vi "Test_Stage_Movement.vi"() -> ()   [LabVIEW 2013]
panel:
  in  "Numeric":dbl
  in  "Serial":i32=90848557
  in  "MG17Motor":refnum<k7>(container)
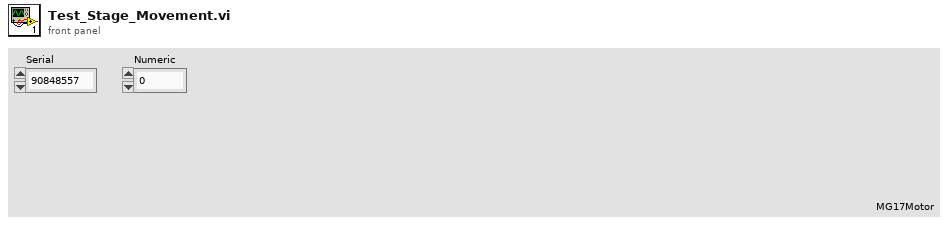
[diagram p1: front panel]
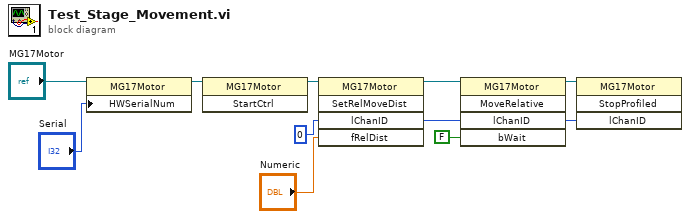
[diagram p0: block diagram]
diagram:
  n1 = property class="MG17Motor"(reference="MG17Motor", "HWSerialNum"="Serial") -> (reference out=w9:refnum<k7>)  [unwired: 1 in, 1 out]
  n2 = invoke class="MG17Motor" method="StartCtrl"(reference=w9) -> (reference out=w3:refnum<k7>)  [unwired: 2 in, 2 out]
  n3 = invoke class="MG17Motor" method="SetRelMoveDist"(reference=w3, "lChanID"=0, "fRelDist"="Numeric") -> (reference out=w7:refnum<k7>, "lChanID"=w6:i32)  [unwired: 2 in, 3 out]
  n4 = invoke class="MG17Motor" method="MoveRelative"(reference=w7, "lChanID"=w6, "bWait"=FALSE) -> (reference out=w5:refnum<k7>, "lChanID"=w4:i32)  [unwired: 2 in, 3 out]
  n5 = invoke class="MG17Motor" method="StopProfiled"(reference=w5, "lChanID"=w4) -> ()  [unwired: 2 in, 4 out]
